vi "Hood Manual.vi"(7 "Description":string, 8 "Command Info In":T1, 11 "Setpoint":dbl) -> (0 "Command Info Out":T1)   [LabVIEW 2025]
doc: "This template is useful for immediate subsystem actions that do not need deadband filtering\n\nBe sure to right-click and select New from Template and save with a new command name."
uses:
  <vilib>/Rock Robotics/WPI/Framework/Command Status Info.ctl
  <vilib>/Rock Robotics/WPI/Framework/Completion Status.ctl
  <vilib>/Rock Robotics/WPI/Framework/Completion Notifier.ctl
  Implementation/Shooter Operations.ctl
  Implementation/Shooter Setpoints.ctl
  swerve-template/Type Definitions/Data/Robot Velocities.ctl
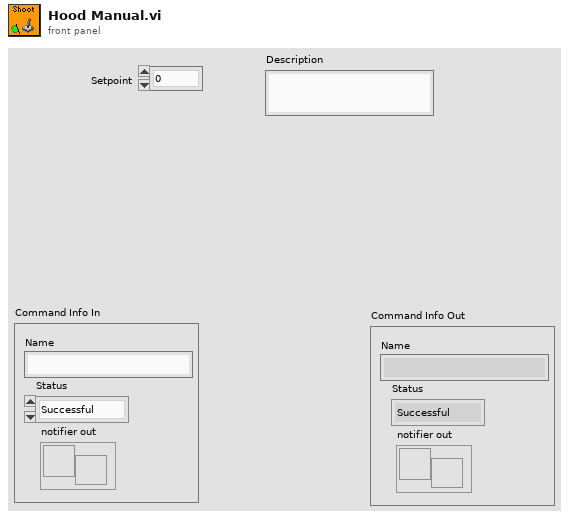
[diagram p1: front panel]
types:
  T1 = typedef "Command Status Info.ctl" = cluster{"Name":string, "Status":T2, "notifier out":T3}
  T2 = typedef "Completion Status.ctl" = enum16{"Successful", "Aborted", "Incomplete"}
  T3 = typedef "Completion Notifier.ctl" = refnum<notifier>
  T4 = typedef "Shooter Operations.ctl" = enum16{"Reserve", "Read Current", "Interpolated Shot", "Hood Manual", "Reset Hood", "Immediate", "Start Popcorn", "Start Shooter"}
  T5 = typedef "Shooter Setpoints.ctl" = cluster{"Operation":T4, "Setpoint":dbl, "Duration":dbl, "Robot Velocities":T6, "Hood Setpoint":dbl}
  T6 = typedef "Robot Velocities.ctl" = cluster{"X Velocity":dbl, "Y Velocity":dbl, "Rotational \nVelocity":dbl}
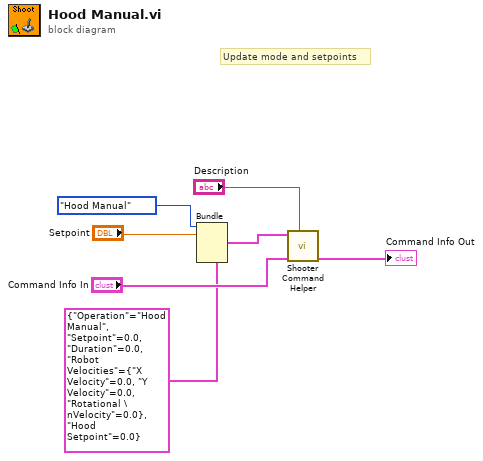
[diagram p0: block diagram]
diagram:
  # "Update mode and setpoints"
  n1 = Bundle(cluster=T5 {"Operation"=enum."Hood Manual", "Setpoint"=0.0, "Duration"=0.0, "Robot Velocities"={"X Velocity"=0.0, "Y Velocity"=0.0, "Rotational \nVelocity"=0.0}, "Hood Setpoint"=0.0} ("SubSystem Data"), "Operation"=Shooter_Operations."Hood Manual", "Setpoint"="Setpoint") -> (w2:T5)  [unwired: 3 in]
  n2 = call "Shooter Command Helper.vi"("Description"="Description", "Command Info In"="Command Info In", "SubSystem Data"=w2) -> ("Command Info Out"=→"Command Info Out":T1)  [unwired: 6 in, 2 out]
